vi "chkIfTblHasSameSec.vi"(9 "rowNumAtWhichSecExist":i32, 10 "Section":string, 11 "tbl":string[][](array[string])) -> (3 "foundSameSec?":bool)   [LabVIEW 2010]
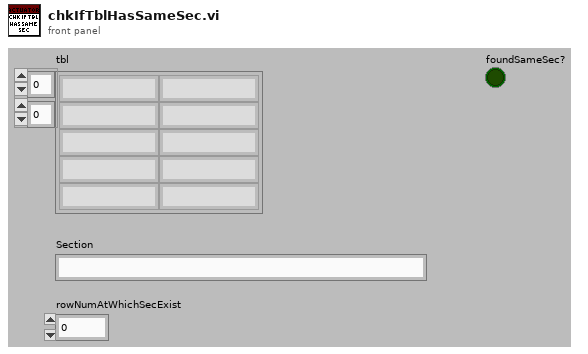
[diagram p1: front panel]
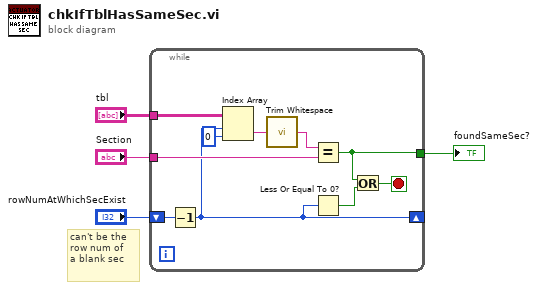
[diagram p0: block diagram]
diagram:
  # "can't be the\nrow num of\na blank sec"
  n1 = while {
    shift-right: [w6] -> _
    shift-left: "rowNumAtWhichSecExist" -> [w7]
    tunnel: "tbl" -> [w14]
    tunnel: "Section" -> [w8]
    tunnel: [w5] -> w1
    stop <- w10 stop-if-true
    n2 = Decrement(x=w7) -> (x-1=w6:i32)
    n3 = Index Array(array=w14, index (row)=w6, index (col)=0 ("disabled index (col)")) -> (element=w12:string)
    n4 = call <vilib>:"Trim Whitespace.vi"("string"=w12) -> ("trimmed string"=w9:string)  [unwired: 1 in]
    n5 = Equal?(x=w9, y=w8) -> (x = y?=w5:bool)
    n6 = Less Or Equal To 0?(x=w6) -> (x <= 0?=w11:bool)
    n7 = Or(x=w5, y=w11) -> (x .or. y?=w10:bool)
  }
  "foundSameSec?" <- w1
